vi "File Parser VI.vi"(8 "error in (no error)":errorcluster, 10 "Original Timing File Path":path, 11 "Perl Parser Path":path) -> (0 "error out":errorcluster, 2 "Parsed File Path":path)   [LabVIEW 2012]
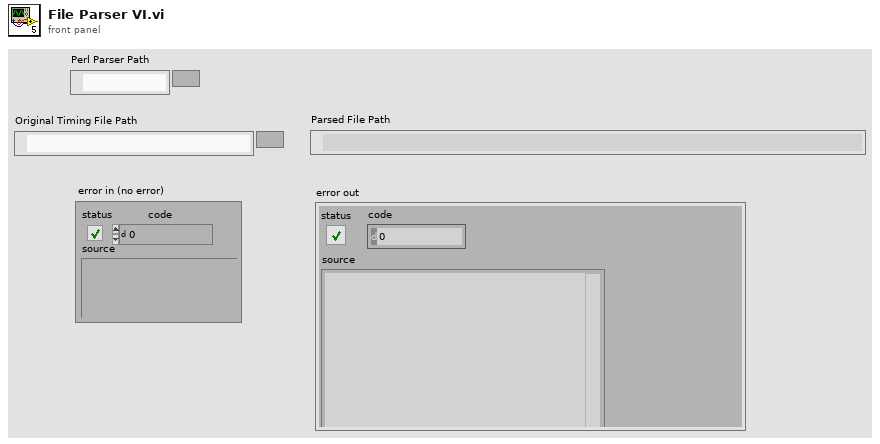
[diagram p1: front panel]
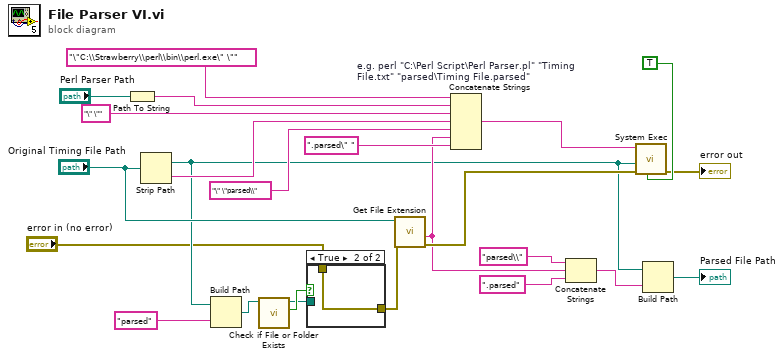
[diagram p0: block diagram]
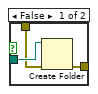
[diagram p2: hidden frame]
diagram:
  n1 = Path To String(path="Perl Parser Path") -> (string=w23:string)
  n2 = Strip Path(path="Original Timing File Path") -> (stripped path=w8:path, name=w22:string)
  n3 = Build Path(base path=w8, name or relative path="parsed") -> (appended path=w6:path)
  n4 = call <vilib>:"Check if File or Folder Exists.vi"("path"=w6) -> ("file or folder exists?"=w5:bool, "dup path"=w4:path)  [unwired: 8 in, 1 out]
  n5 = case shown="True" w5 {
    tunnel: w4 -> [w27 _]
    tunnel: "error in (no error)" -> [w26 w28]
    tunnel: [w25 w28] -> w2
    frame False {
      n6 = Create Folder(path (use dialog)=w27, error in=w26) -> (error out=w25:errorcluster)  [unwired: 1 in, 2 out]
    }
    frame True {
    }
  }
  n7 = call <vilib>:"Get File Extension.vi"("error in (no error)"=w2, "file"="Original Timing File Path") -> ("error out"=w19:errorcluster, "filename without extension"=w18:string)  [unwired: 6 in, 2 out]
  n8 = Concatenate Strings "e.g. perl \"C:\\Perl Script\\Perl Parser.pl\" \"Timing File.txt\" \"parsed\\Timing File.parsed\""("\"C:\\Strawberry\\perl\\bin\\perl.exe\" \"", w23, "\" \"", w22, "\" \"parsed\\", w18, ".parsed\" ") -> (w1:string)
  n9 = Concatenate Strings("parsed\\", w18, ".parsed") -> (w11:string)
  n10 = call <vilib>:"System Exec.vi"("run minimized? (F)"=TRUE, "error in (no error)"=w19, "working directory"=w8, "command line"=w1) -> ("error out"=→"error out":errorcluster)  [unwired: 4 in, 3 out]
  n11 = Build Path(base path=w8, name or relative path=w11) -> (appended path=→"Parsed File Path":path)
